vi "cw_2_2.vi"() -> ()   [LabVIEW 2022 SP3]
uses:
  <vilib>/numeric/Random Number (Range) DBL.vi
panel:
  out "LED":bool
  in  "discrimination level":dbl=1.0 step=0.1
  in  "noise amplitude":ext=0.5
  out "Waveform Chart":cluster{dbl, "discrimination level":dbl}(graph)
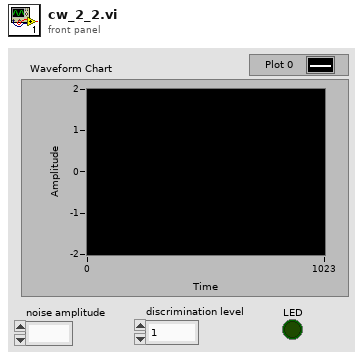
[diagram p1: front panel]
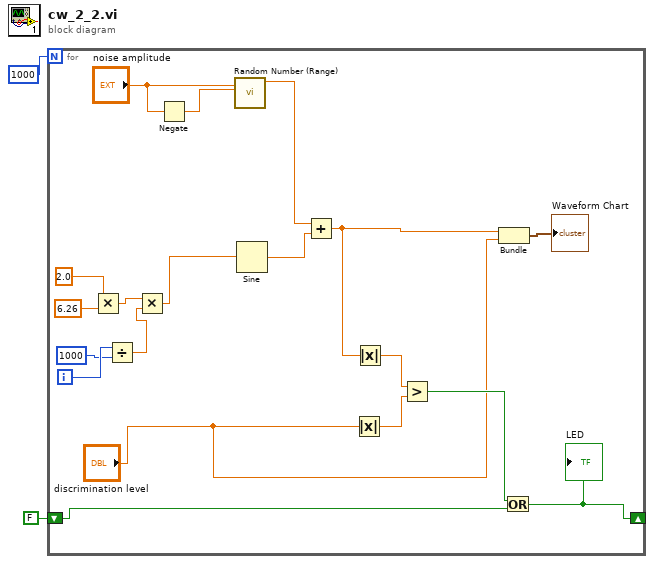
[diagram p0: block diagram]
diagram:
  n1 = for {
    N: 1000 -> [_]
    shift-right: [w4] -> _
    shift-left: FALSE -> [w6]
    i -> [w20]
    n2 = Multiply(x=2.0, y=6.26) -> (x*y=w18:dbl)
    n3 = Divide(x=w20, y=1000) -> (x/y=w17:dbl)
    n4 = Multiply(x=w18, y=w17) -> (x*y=w16:dbl)
    n5 = Negate(x="noise amplitude") -> (-x=w12:ext)
    n6 = call-poly <vilib>:"Random Number (Range).vi"("lower bound (0)"=w12, "upper bound (100)"="noise amplitude") -> ("number"=w14:dbl)  [unwired: 9 in]
    n7 = Sine(x=w16) -> (sin(x)=w15:dbl)
    n8 = Add(x=w14, y=w15) -> (x+y=w9:dbl)
    n9 = Absolute Value(x="discrimination level") -> (abs(x)=w7:dbl)
    n10 = Absolute Value(x=w9) -> (abs(x)=w8:dbl)
    n11 = Greater?(x=w8, y=w7) -> (0:w5:bool)
    n12 = Bundle(w9, "discrimination level"="discrimination level") -> (→"Waveform Chart":cluster{dbl, "discrimination level":dbl})  [unwired: 1 in]
    n13 = Or(x=w5, y=w6) -> (x .or. y?=w4:bool)
    "LED" <- w4
  }
